vi "sub_state_fgv.vi"(7 "cmd":enum16{"read", "write"}(ring), 11 "Initial States":T1=[0.0, 0.0, 0.0, 0.0] format="%.4f") -> (3 "state_out":dbl[](array[numeric]))   [LabVIEW 2018]
uses:
  Model/States.ctl
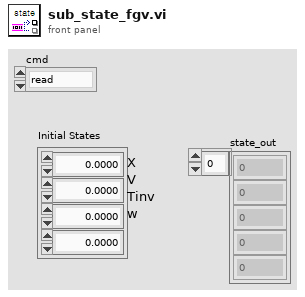
[diagram p1: front panel]
types:
  T1 = typedef "States.ctl" = dbl[]
  T2 = typedef "ctr-ref.ctl" = cluster{"connected":refnum<vi>, "start":refnum<vi>, "read_data":refnum<vi>, "Target":refnum<vi>, "play_type":refnum<vi>, "dt_daq":refnum<vi>, "dt_tcp":refnum<vi>, "timer":refnum<vi>, "States":refnum<vi>, "angle_limit":refnum<vi>, "Initial States":refnum<vi>}
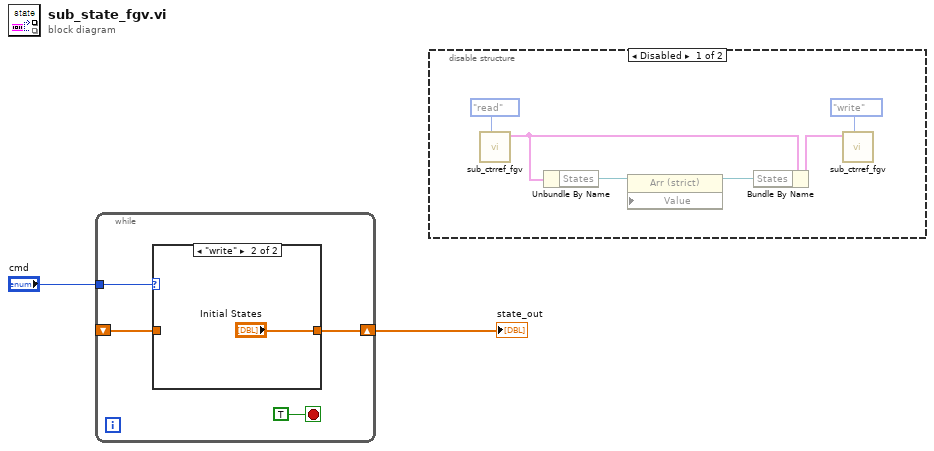
[diagram p0: block diagram]
diagram:
  n1 = while {
    tunnel: "cmd" -> [w5]
    shift-right: [w4] -> w1
    shift-left: _ -> [w3]
    stop <- TRUE stop-if-true
    n2 = case shown="\"write\"" w5 {
      tunnel: [w7 "Initial States"] -> w4
      tunnel: w3 -> [w7 _]
      frame "read", Default {
      }
      frame "write" {
      }
    }
  }
  "state_out" <- w1
  n3 = disable-structure shown="Disabled" {
    frame Disabled {
      n4 = call "sub_ctrref_fgv.vi"("cmd"=enum16{"write", "read"}."read") -> ("ctr_out"=w13:T2)  [unwired: 10 in]
      n5 = Unbundle By Name(w13) -> ("States"=w12:refnum<vi>)
      n6 = property class="Arr (strict)" props=["Value"](reference=w12) -> (reference out=w11:refnum<vi>)  [unwired: 2 in, 1 out]
      n7 = Bundle By Name(cluster=w13, "States"=w11) -> (w9:T2)
      n8 = call "sub_ctrref_fgv.vi"("cmd"=enum16{"write", "read"}."write", "ctr_in"=w9) -> ()  [unwired: 9 in, 1 out]
    }
    frame Enabled {
    }
  }
